vi "Auto Loop.vi"(8 "error in":errorcluster, 10 "semaphore":T3, 11 "Queues in":T10) -> (0 "error out":errorcluster, 2 "semaphore out":T3)   [LabVIEW 2017]
doc: "This is the loop that handles the testing algorithms\n\n--------------\nv0.1:\n\n- Updated Printer"
uses:
  support/Message Queue/All Message Queues.ctl
  support/Message Queue/Message Cluster.ctl
  controls/Model Name.ctl
  controls/Auto States v0.2.ctl
  controls/All Specs.ctl
  controls/Specifications.ctl
  controls/Results Cluster.ctl
  controls/AC Results.ctl
  controls/Update Measurements.ctl
  <vilib>/Platform/TimedLoop/XDataNode/timing_clust.ctl
  <vilib>/Platform/TimedLoop/XDataNode/nitl_modes.ctl
  <vilib>/Platform/TimedLoop/XDataNode/wakeup.ctl
  controls/Towerlight.ctl
  support/Message Queue/Enqueue Message (Single).vi
  GV/All Inputs.vi
  support/GV/Towerlight GV.vi
  GV/TEST GV/Test auto state machine.vi
  <vilib>/platform/TimedLoop/XDataNode/XDataNode.xnode
  controls/FGV DO.ctl
  <vilib>/Platform/TimedLoop/XDataNode/XDNodeRunTimeDep.lvlib
  support/Message Queue/Message Queue.lvlib
panel:
  out "Results 2":T1
  out "TS Status 2":cluster{"Status":string, "Elapsed Time":dbl}
  out "Results Cluster out 2":T2
  out "Graph 2":dbl[][](array[numeric])
  out "cycle time 2":u32
  out "Specs":T4={"LH"={"Go Up"={"Min Speed"=120.0, "Max Speed"=10.0, "Min Time"=1.82, "Max Time"=3.7, "Min Run Current"=0.0, "Max Run Current"=10.0, "Min Stall Current"=0.0, "Max Stall Current"=25.0, "Min Stall Force"=170.0, "Max Stall Force"=320.0, "Min Stroke"=170.0, "Max Stroke"=320.0}, "Go Down"={"Min Speed"=10.0, "Max Speed"=250.0, "Min Travel Time"=1.82, "Max Travel Time"=3.7, "Min Run Current"=0.0, "Max Run Current"=10.0}, "Shipping"={"Min Distance"=150.0, "Max Distance"=300.0, "Setpoint"=5.0}, "Anti-Pinch"={"Min Force"=5.0, "Max Force"=15.0}}, "RH"={"Go Up"={"Min Speed"=120.0, "Max Speed"=10.0, "Min Time"=1.82, "Max Time"=3.7, "Min Run Current"=0.0, "Max Run Current"=10.0, "Min Stall Current"=0.0, "Max Stall Current"=25.0, "Min Stall Force"=170.0, "Max Stall Force"=320.0, "Min Stroke"=170.0, "Max Stroke"=320.0}, "Go Down"={"Min Speed"=10.0, "Max Speed"=250.0, "Min Travel Time"=1.82, "Max Travel Time"=3.7, "Min Run Current"=0.0, "Max Run Current"=10.0}, "Shipping"={"Min Distance"=150.0, "Max Distance"=300.0, "Setpoint"=5.0}, "Anti-Pinch"={"Min Force"=5.0, "Max Force"=15.0}}, "W 601 FR RH Std"={"Go Up"={"Min Speed"=10.0, "Max Speed"=250.0, "Min Time"=0.5, "Max Time"=4.3, "Min Run Current"=0.0, "Max Run Current"=10.0, "Min Stall Current"=0.0, "Max Stall Current"=25.0, "Min Stall Force"=170.0, "Max Stall Force"=320.0, "Min Stroke"=254.4, "Max Stroke"=270.4}, "Go Down"={"Min Speed"=10.0, "Max Speed"=250.0, "Min Travel Time"=0.5, "Max Travel Time"=4.3, "Min Run Current"=0.0, "Max Run Current"=10.0}, "Shipping"={"Min Distance"=5.0, "Max Distance"=15.0, "Setpoint"=5.0}, "Anti-Pinch"={"Min Force"=5.0, "Max Force"=15.0}}, "W 601 FR LH Std"={"Go Up"={"Min Speed"=10.0, "Max Speed"=250.0, "Min Time"=0.5, "Max Time"=4.3, "Min Run Current"=0.0, "Max Run Current"=10.0, "Min Stall Current"=0.0, "Max Stall Current"=25.0, "Min Stall Force"=170.0, "Max Stall Force"=320.0, "Min Stroke"=254.4, "Max Stroke"=270.4}, "Go Down"={"Min Speed"=10.0, "Max Speed"=250.0, "Min Travel Time"=0.5, "Max Travel Time"=4.3, "Min Run Current"=0.0, "Max Run Current"=10.0}, "Shipping"={"Min Distance"=5.0, "Max Distance"=15.0, "Setpoint"=5.0}, "Anti-Pinch"={"Min Force"=5.0, "Max Force"=15.0}}, "W 601 RR RH Std"={"Go Up"={"Min Speed"=10.0, "Max Speed"=250.0, "Min Time"=0.5, "Max Time"=4.3, "Min Run Current"=0.0, "Max Run Current"=10.0, "Min Stall Current"=0.0, "Max Stall Current"=25.0, "Min Stall Force"=170.0, "Max Stall Force"=320.0, "Min Stroke"=254.4, "Max Stroke"=270.4}, "Go Down"={"Min Speed"=10.0, "Max Speed"=250.0, "Min Travel Time"=0.5, "Max Travel Time"=4.3, "Min Run Current"=0.0, "Max Run Current"=10.0}, "Shipping"={"Min Distance"=5.0, "Max Distance"=15.0, "Setpoint"=5.0}, "Anti-Pinch"={"Min Force"=5.0, "Max Force"=15.0}}, "W 601 RR LH Std"={"Go Up"={"Min Speed"=10.0, "Max Speed"=250.0, "Min Time"=0.5, "Max Time"=4.3, "Min Run Current"=0.0, "Max Run Current"=10.0, "Min Stall Current"=0.0, "Max Stall Current"=25.0, "Min Stall Force"=170.0, "Max Stall Force"=320.0, "Min Stroke"=254.4, "Max Stroke"=270.4}, "Go Down"={"Min Speed"=10.0, "Max Speed"=250.0, "Min Travel Time"=0.5, "Max Travel Time"=4.3, "Min Run Current"=0.0, "Max Run Current"=10.0}, "Shipping"={"Min Distance"=5.0, "Max Distance"=15.0, "Setpoint"=5.0}, "Anti-Pinch"={"Min Force"=5.0, "Max Force"=15.0}}, "W 601 FR RH AP"={"Go Up"={"Min Speed"=10.0, "Max Speed"=250.0, "Min Time"=0.5, "Max Time"=4.3, "Min Run Current"=0.0, "Max Run Current"=10.0, "Min Stall Current"=0.0, "Max Stall Current"=25.0, "Min Stall Force"=170.0, "Max Stall Force"=320.0, "Min Stroke"=254.4, "Max Stroke"=270.4}, "Go Down"={"Min Speed"=10.0, "Max Speed"=250.0, "Min Travel Time"=0.5, "Max Travel Time"=4.3, "Min Run Current"=0.0, "Max Run Current"=10.0}, "Shipping"={"Min Distance"=5.0, "Max Distance"=15.0, "Setpoint"=5.0}, "Anti-Pinch"={"Min Force"=5.0, "Max Force"=15.0}}, "W 601 FR LH AP"={"Go Up"={"Min Speed"=10.0, "Max Speed"=250.0, "Min Time"=0.5, "Max Time"=4.3, "Min Run Current"=0.0, "Max Run Current"=10.0, "Min Stall Current"=0.0, "Max Stall Current"=25.0, "Min Stall Force"=170.0, "Max Stall Force"=320.0, "Min Stroke"=254.4, "Max Stroke"=270.4}, "Go Down"={"Min Speed"=10.0, "Max Speed"=250.0, "Min Travel Time"=0.5, "Max Travel Time"=4.3, "Min Run Current"=0.0, "Max Run Current"=10.0}, "Shipping"={"Min Distance"=5.0, "Max Distance"=15.0, "Setpoint"=5.0}, "Anti-Pinch"={"Min Force"=5.0, "Max Force"=15.0}}, "W 601 RR RH AP"={"Go Up"={"Min Speed"=10.0, "Max Speed"=250.0, "Min Time"=0.5, "Max Time"=4.3, "Min Run Current"=0.0, "Max Run Current"=10.0, "Min Stall Current"=0.0, "Max Stall Current"=25.0, "Min Stall Force"=170.0, "Max Stall Force"=320.0, "Min Stroke"=254.4, "Max Stroke"=270.4}, "Go Down"={"Min Speed"=10.0, "Max Speed"=250.0, "Min Travel Time"=0.5, "Max Travel Time"=4.3, "Min Run Current"=0.0, "Max Run Current"=10.0}, "Shipping"={"Min Distance"=5.0, "Max Distance"=15.0, "Setpoint"=5.0}, "Anti-Pinch"={"Min Force"=5.0, "Max Force"=15.0}}, "W 601 RR LH AP"={"Go Up"={"Min Speed"=10.0, "Max Speed"=250.0, "Min Time"=0.5, "Max Time"=4.3, "Min Run Current"=0.0, "Max Run Current"=10.0, "Min Stall Current"=0.0, "Max Stall Current"=25.0, "Min Stall Force"=170.0, "Max Stall Force"=320.0, "Min Stroke"=254.4, "Max Stroke"=270.4}, "Go Down"={"Min Speed"=10.0, "Max Speed"=250.0, "Min Travel Time"=0.5, "Max Travel Time"=4.3, "Min Run Current"=0.0, "Max Run Current"=10.0}, "Shipping"={"Min Distance"=5.0, "Max Distance"=15.0, "Setpoint"=5.0}, "Anti-Pinch"={"Min Force"=5.0, "Max Force"=15.0}}}
  out "Counts":T6
  out "AC State":T7
  in  "Initial Data":T9={"Model Name"=enum."W 501 FLH Std.", "ID"="ID", "Shift"=""}
  in  "Exit":bool
  out "Period":i64
  in  "Run Auto?":bool
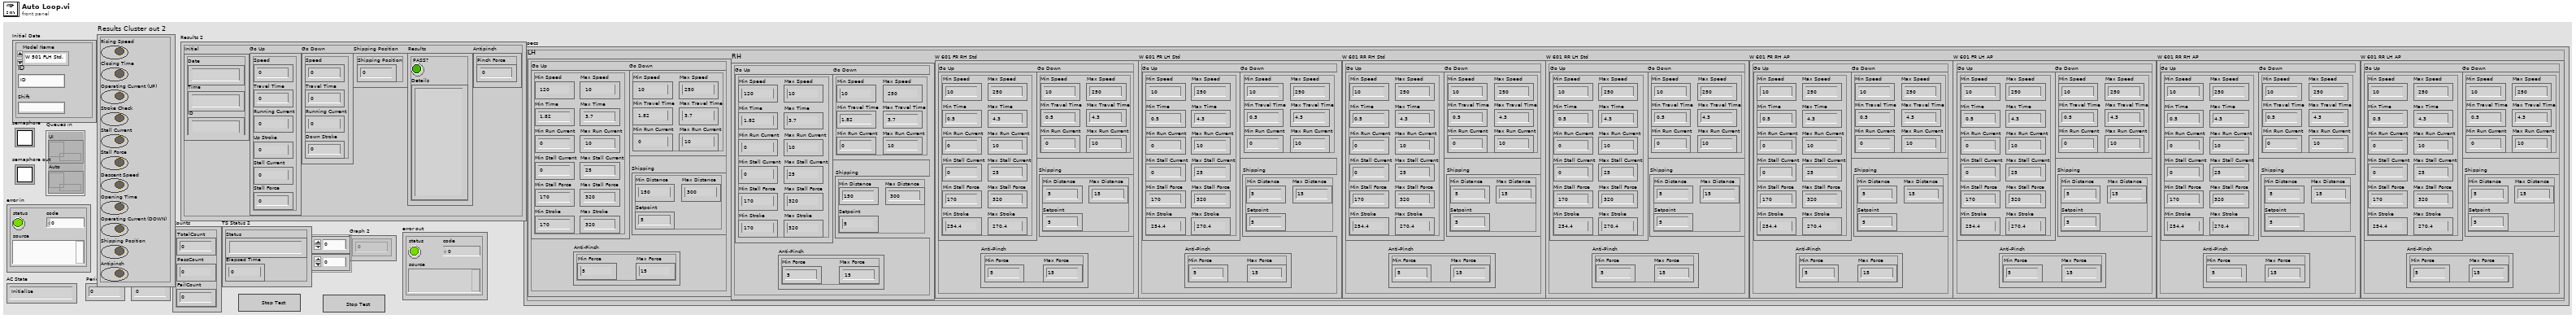
[diagram p1: front panel]
types:
  T1 = typedef "AC Results.ctl" = cluster{"Initial":cluster{"Date":string, "Time":string, "ID":string}, "Go Up":cluster{"Speed":dbl, "Travel Time":dbl, "Running Current":dbl, "Up Stroke":dbl, "Stall Current":dbl, "Stall Force":dbl}, "Go Down":cluster{"Speed":dbl, "Travel Time":dbl, "Running Current":dbl, "Down Stroke":dbl}, "Shipping Position":cluster{"Shipping Position":dbl}, "Results":cluster{"PASS?":bool, "Details":string}, "Antipinch":cluster{"Pinch Force":dbl}}
  T2 = typedef "Results Cluster.ctl" = cluster{"Rising Speed":bool, "Closing Time":bool, "Operating Current (UP)":bool, "Stroke Check":bool, "Stall Current":bool, "Stall Force":bool, "Descent Speed":bool, "Opening Time":bool, "Operating Current (DOWN)":bool, "Shipping Position":bool, "Antipinch":bool}
  T3 = typedef "Semaphore RefNum" = refnum<k1>
  T4 = typedef "All Specs.ctl" = cluster{"LH":T5, "RH":T5, "W 601 FR RH Std":T5, "W 601 FR LH Std":T5, "W 601 RR RH Std":T5, "W 601 RR LH Std":T5, "W 601 FR RH AP":T5, "W 601 FR LH AP":T5, "W 601 RR RH AP":T5, "W 601 RR LH AP":T5}
  T5 = typedef "Specifications.ctl" = cluster{"Go Up":cluster{"Min Speed":dbl, "Max Speed":dbl, "Min Time":dbl, "Max Time":dbl, "Min Run Current":dbl, "Max Run Current":dbl, "Min Stall Current":dbl, "Max Stall Current":dbl, "Min Stall Force":dbl, "Max Stall Force":dbl, "Min Stroke":dbl, "Max Stroke":dbl}, "Go Down":cluster{"Min Speed":dbl, "Max Speed":dbl, "Min Travel Time":dbl, "Max Travel Time":dbl, "Min Run Current":dbl, "Max Run Current":dbl}, "Shipping":cluster{"Min Distance":dbl, "Max Distance":dbl, "Setpoint":dbl}, "Anti-Pinch":cluster{"Min Force":dbl, "Max Force":dbl}}
  T6 = cluster{"TotalCount":u16, "PassCount":u16, "FailCount":u16}
  T7 = typedef "Auto States v0.2.ctl" = enum16{"Initialize", "Check Pressure", "Check EStop", "Check Reject Door ", "Check ReadyCondition", "Wait to Home", "Declamping", "Loadcell CYL to Home", "Wait for Part Presence", "Wait for Hands-Off", "Clamp", "Wait for Load Engage", "Wait for Start", "Test Sequencer", "Log & Print", "check for pass or fail", "Result", "Wait for Reject Door Open", "Wait for Reject 2 OFF", "Wait for Reject 2 ON", "Wait for Reject 1 OFF", "Wait for Reject 1 ON", "Wait for Reject Door Close"}
  T8 = typedef "Model Name.ctl" = enum16{"W 501 FLH Std.", "W 501 FRH Std.", "W 601 FR RH Std", "W 601 FR LH Std", "W 601 RR RH Std", "W 601 RR LH Std", "W 601 FR RH AP", "W 601 FR LH AP", "W 601 RR RH AP", "W 601 RR LH AP"}
  T9 = cluster{"Model Name":T8, "ID":string, "Shift":string}
  T10 = typedef "Message Queue.lvlib/All Message Queues.ctl" = cluster{"UI":refnum<queue>, "Auto":refnum<queue>}
  T11 = cluster{"AI":refnum<k21>, "DI":refnum<k21>, "Counter":refnum<k21>}
  T12 = typedef "Towerlight.ctl" = enum16{"Idle", "Error", "Attention", "Running", "Maintenance", "Fail"}
  T13 = typedef "FGV DO.ctl" = enum16{"Initialize", "Start Task", "Clamping", "Load CYL", "Contactors", "Loadcell CYL", "BSL", "Read DO", "Clear Tasks", "Clear Task"}
  T14 = typedef "XDNodeRunTimeDep.lvlib/timing_clust.ctl" = cluster{"Expected End [f-1]":u64, "Actual End [f-1]":u64, "Finished Late? [f-1]":bool, "Expected End [i-1]":u64, "Actual End [i-1]":u64, "Finished Late? [i-1]":bool, "Expected Start [i]":u64, "Actual Start [i]":u64, "Expected Start [f]":u64, "Actual Start [f]":u64, "Source Name":string, "Structure Name":string, "Period":i64, "Deadline":i64, "Offset":i64, "Start":i64, "Priority":i32, "Timeout":i32, "Mode":T15, "Wakeup Reason":T16, "Error":errorcluster, "Source Type":string, "Secondary Source Type":string, "Global End Time":u64, "Global Start Time":u64, "Frame Duration":u64, "Iteration Duration":u64, "Assigned CPU":i32, "I/O Scan Engine Mode":u32}
  T15 = typedef "XDNodeRunTimeDep.lvlib/nitl_modes.ctl" = enum32{"No Change", "Process missed periods, maintain original phase", "Discard missed periods, maintain original phase", "Process missed periods, ignore original phase", "Discard missed periods, ignore original phase"}
  T16 = typedef "XDNodeRunTimeDep.lvlib/wakeup.ctl" = enum32{"Normal", "Aborted", "Asynchronous wakeup", "Timing source error", "Timed loop error", "Timeout"}
  T17 = typedef "All Inputs.ctl" = cluster{"DI":cluster{"Machine ON":bool, "E-Stop":bool, "Pressure":bool, "Start":bool, "Safety Curtain":bool, "RS Load UP Rear":bool, "RS Load UP Front":bool, "RS Load DN Rear":bool, "RS Load DN Front":bool, "RS Loadcell Rear":bool, "RS Loadcell Front":bool, "Reject Sensor 1":bool, "Reject Sensor 2":bool, "Door SW Reject":bool}, "AI":cluster{"Force":dbl[], "Stroke":dbl[], "CurrentMon":dbl[]}, "SACB Inputs":T18}
  T18 = typedef "SACB DI.ctl" = cluster{"RS ClampTop Front":bool, "RS ClampBottom Front":bool, "RS ClampMotorLH Front":bool, "RS ClampMotorRH Front":bool, "IPS PartPresenceTop LH":bool, "IPS PartPresenceBottom LH":bool, "IPS PartPresenceTop RH":bool, "IPS PartPresenceBottom RH":bool, "IPS LoadEngaged 1":bool, "IPS LoadEngaged 2":bool, "IPS LoadEngaged 3":bool, "C11":bool, "C12":bool, "C13":bool, "C14":bool, "C15":bool}
  T19 = cluster{"Pressure":bool, "E Stop":bool, "Reject Door":bool, "Ready Condition":bool, " Home":bool, " De Clamb":bool, " Load Cell":bool, " Part Presence":bool, " Hands Off":bool, "Clamp":bool, " Load engage":bool, "Wait Start":bool, "Test Sequencer":bool}
  T20 = typedef "Update Measurements.ctl" = cluster{"Results":T1, "TS Status":cluster{"Status":string, "Elapsed Time":dbl}, "Counts":cluster{"TotalCount":u16, "PassCount":u16, "FailCount":u16}, "AC Graph":cluster{"X":dbl, "Y":dbl}[], "Total Time":dbl, "Testing Time (s)":dbl, "Graph":dbl[][], "signal out":waveform(dbl)}
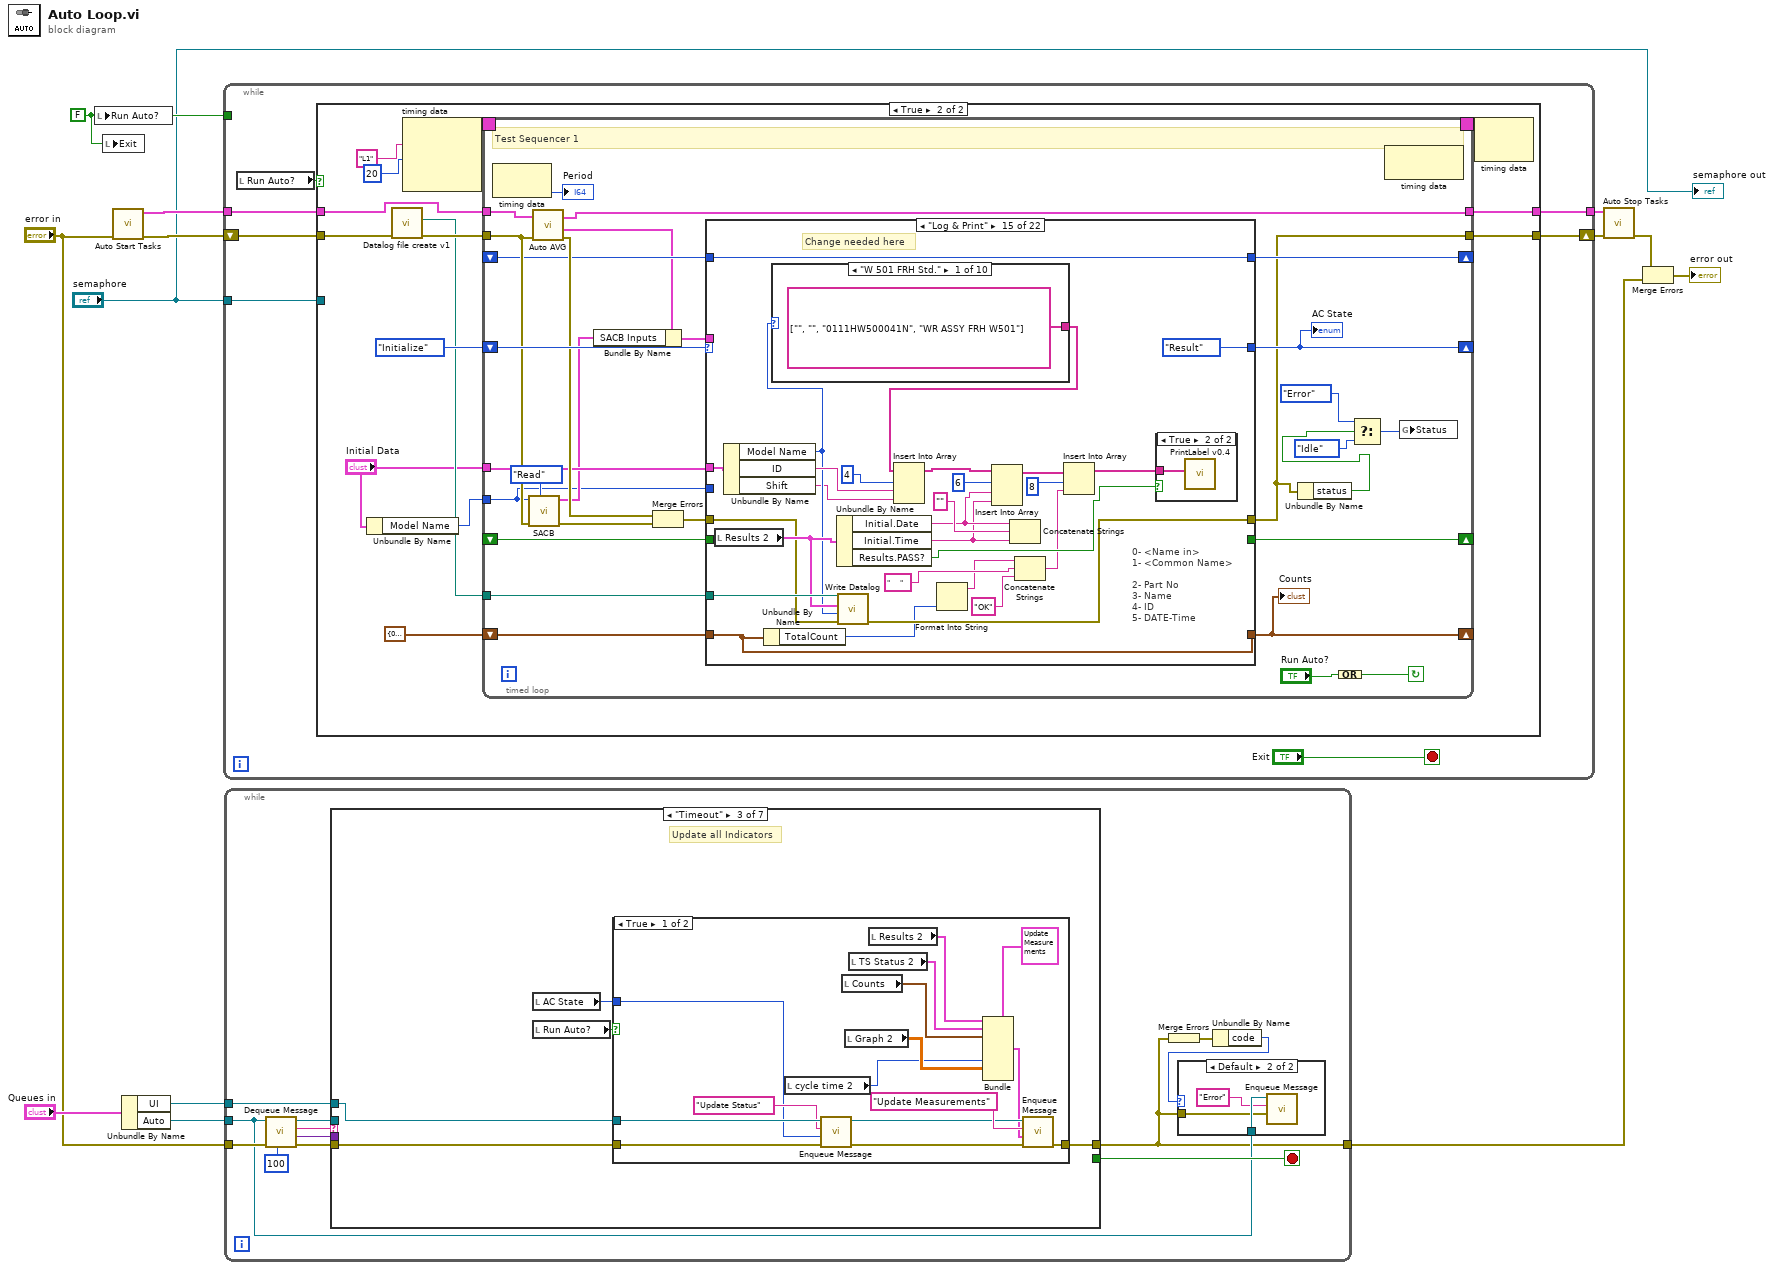
[diagram p0: block diagram]
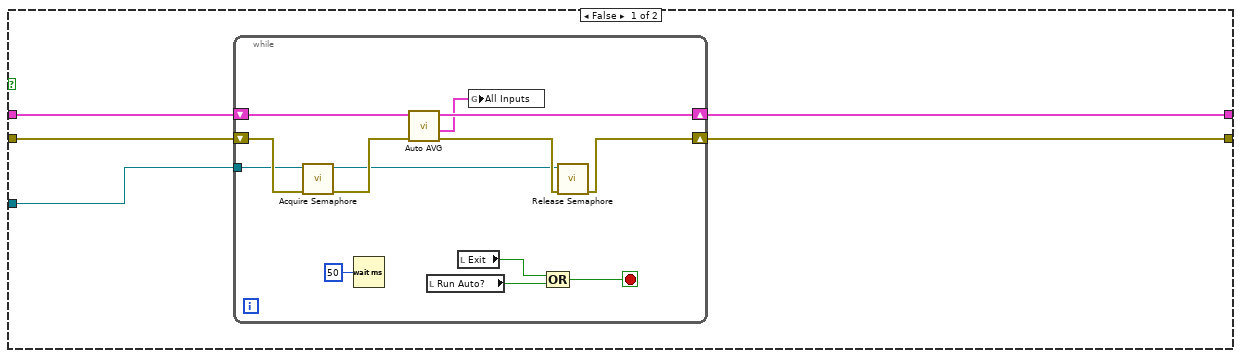
[diagram p2: hidden frame]
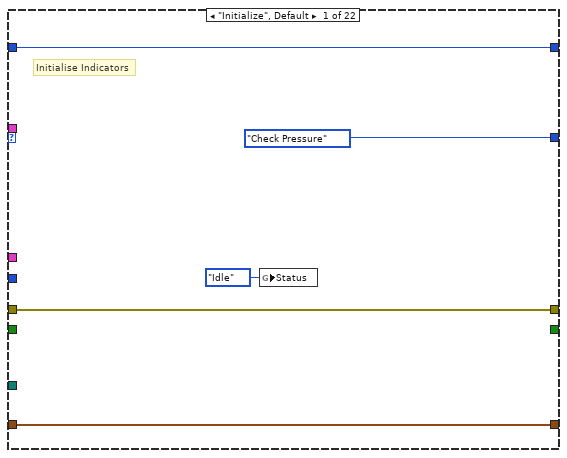
[diagram p3: hidden frame]
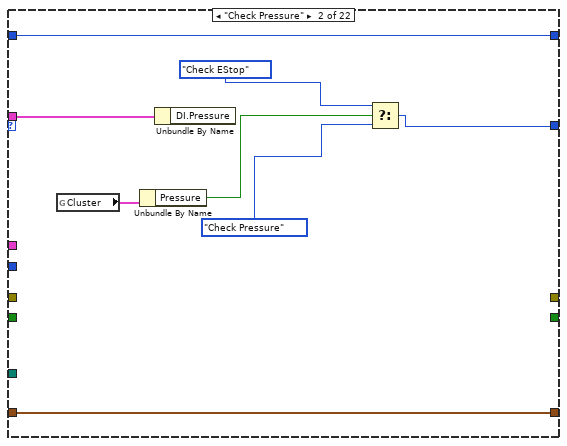
[diagram p4: hidden frame]
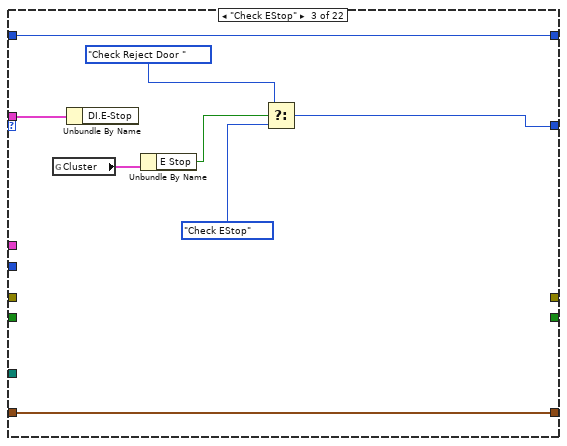
[diagram p5: hidden frame]
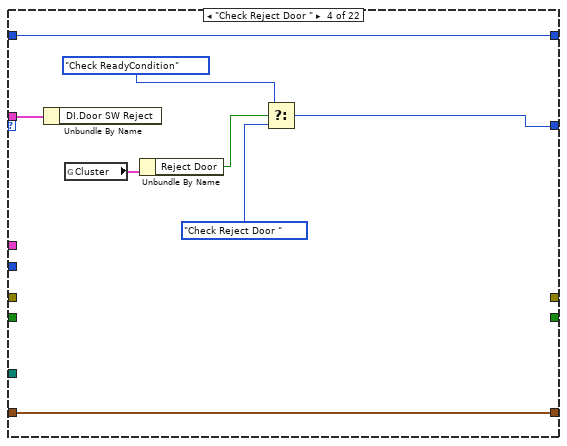
[diagram p6: hidden frame]
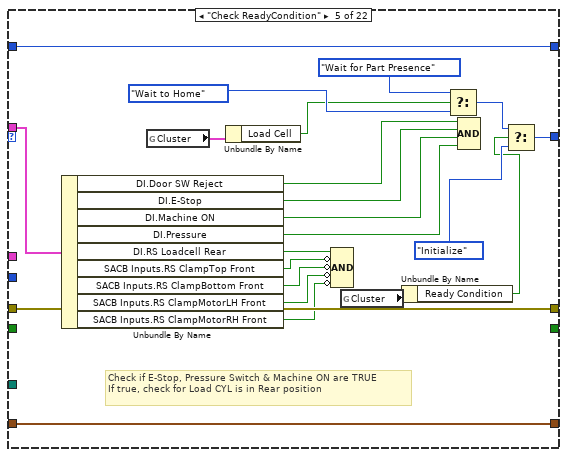
[diagram p7: hidden frame]
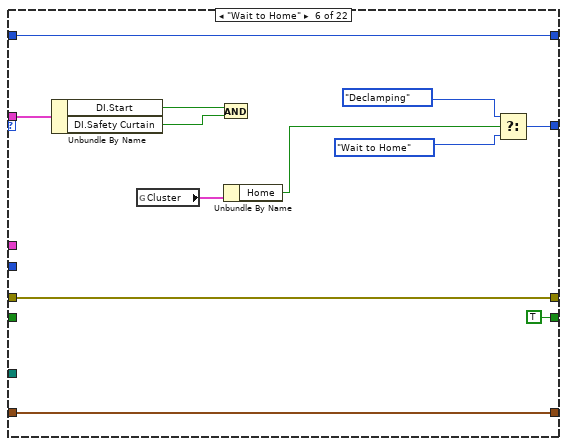
[diagram p8: hidden frame]
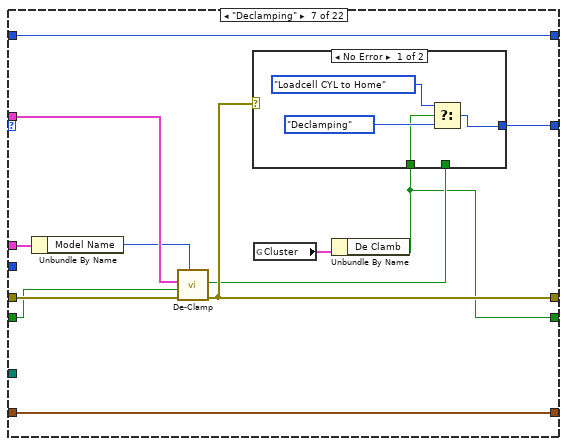
[diagram p9: hidden frame]
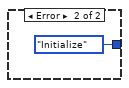
[diagram p10: hidden frame]
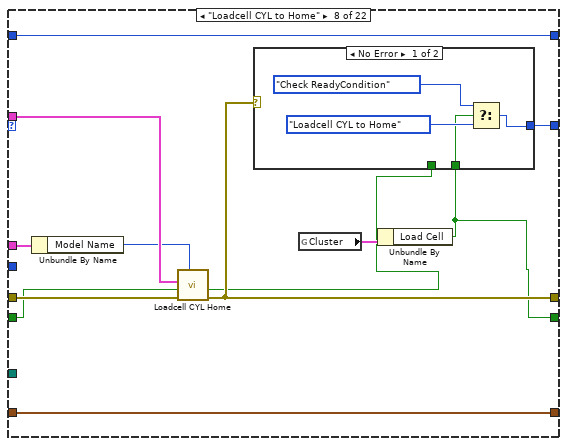
[diagram p11: hidden frame]
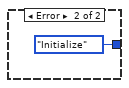
[diagram p12: hidden frame]
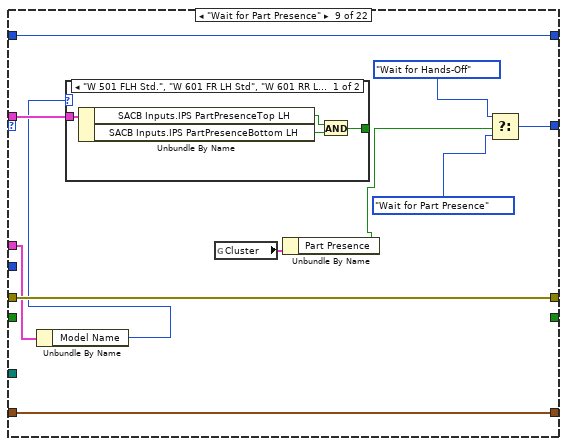
[diagram p13: hidden frame]
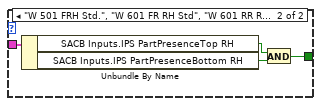
[diagram p14: hidden frame]
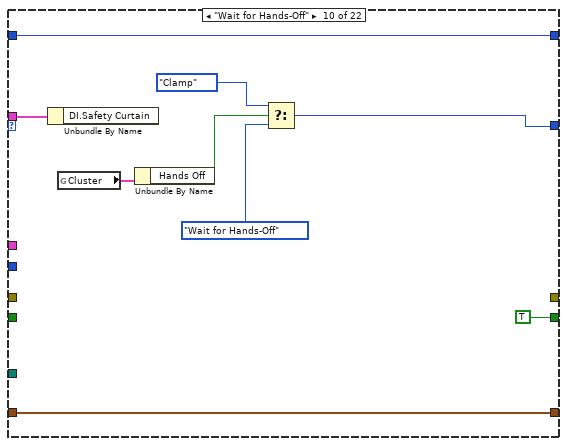
[diagram p15: hidden frame]
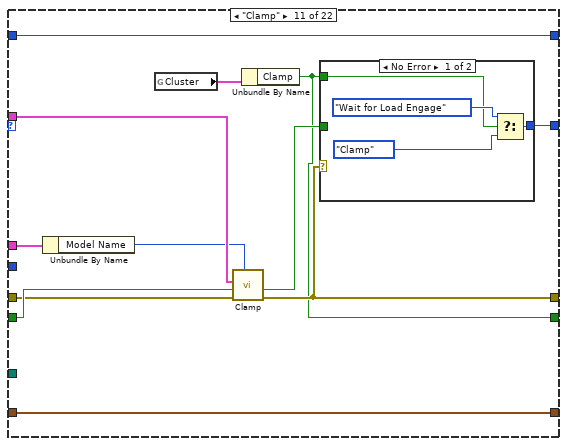
[diagram p16: hidden frame]
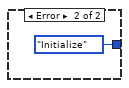
[diagram p17: hidden frame]
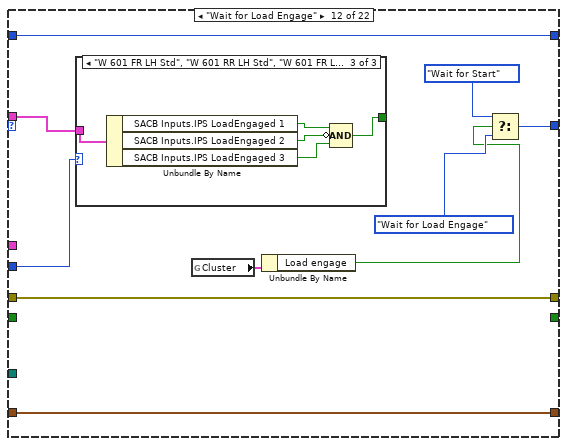
[diagram p18: hidden frame]
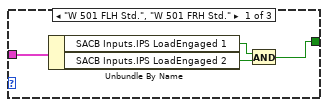
[diagram p19: hidden frame]
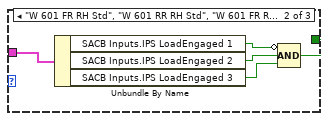
[diagram p20: hidden frame]
diagram:
  w8 = FALSE ("Run Auto?")
  n1 = local write "Run Auto?"(w8) -> ()
  n2 = local write "Exit"(w8) -> ()
  n3 = call "Auto Start Tasks.vi"("error in"="error in") -> ("error out"=w6:errorcluster, "All Input Tasks"=w7:T11)  [unwired: 9 in]
  n4 = Unbundle By Name("Queues in") -> ("UI"=w9:refnum<queue>, "Auto"=w12:refnum<queue>)
  n5 = while {
    shift-right: [w15] -> w3
    shift-left: w6 -> [w17]
    tunnel: w8 -> [_]
    tunnel: w7 -> [w18]
    tunnel: [w16] -> w5
    tunnel: "semaphore" -> [w14]
    stop <- "Exit" stop-if-true
    n6 = local read "Run Auto?"() -> (w19:bool)
    n7 = case shown="True" w19 {
      tunnel: [w23 w43] -> w15
      tunnel: w17 -> [w24 w41]
      tunnel: w18 -> [w25 w44]
      tunnel: [w22 w42] -> w16
      tunnel: w14 -> [w21 _]
      frame False {
        n8 = while {
          shift-right: [w36] -> w22
          shift-left: w25 -> [w37]
          shift-right: [w28] -> w23
          shift-left: w24 -> [w31]
          tunnel: w21 -> [w26]
          stop <- w34 stop-if-true
          n9 = call <vilib>:"Acquire Semaphore.vi"("error in (no error)"=w31, "semaphore"=w26) -> ("error out"=w30:errorcluster, "semaphore out"=w27:T3)  [unwired: 3 in, 1 out]
          n10 = Wait (ms)(milliseconds to wait=u32 50) -> ()  [unwired: 1 out]
          n11 = call "Auto AVG.vi"("error in"=w30, "All Input Tasks in"=w37) -> ("error out"=w29:errorcluster, "All Inputs cluster"=w32:T17, "All Input Tasks out"=w36:T11)  [unwired: 7 in]
          n12 = local read "Run Auto?"() -> (w35:bool)
          n13 = local read "Exit"() -> (w33:bool)
          n14 = global write "All Inputs.vi" "All Inputs"(w32) -> ()
          n15 = Compound Arithmetic op=OR(w33, w35) -> (w34:bool)
          n16 = call <vilib>:"Release Semaphore.vi"("error in (no error)"=w29, "semaphore"=w27) -> ("error out"=w28:errorcluster)  [unwired: 4 in, 1 out]
        }
      }
      frame True {
        n17 = Unbundle By Name("Initial Data") -> ("Model Name"=w39:T8)
        n18 = call "Datalog file create v1.vi"("error in (no error)"=w41) -> ("error out"=w46:errorcluster, "File path out"=w45:path)  [unwired: 9 in]
        n19 = node-c288("L1" ("Structure Name"), i64 20 ("Period")) -> (w52:T14)  [unwired: 1 in]
        n20 = timed-loop {
          timing: w52 -> [_]
          timing-out: [_] -> w51
          tunnel: [w54] -> w42
          shift-right: [w76] -> _
          shift-left: Auto_States_v0.2."Initialize" -> [w77]
          tunnel: [w61] -> w43
          tunnel: "Initial Data" -> [w72]
          shift-right: [w73] -> _
          shift-left: _ -> [w74]
          shift-right: [w70] -> _
          shift-left: T6 {"TotalCount"=0, "PassCount"=0, "FailCount"=0} ("Counts") -> [w71]
          tunnel: w45 -> [w69]
          tunnel: w46 -> [w67]
          tunnel: w44 -> [w68]
          shift-right: [w63] -> _
          shift-left: _ -> [w62]
          tunnel: w39 -> [w53]
          stop <- w80 continue-if-true
          # "Test Sequencer 1"
          n21 = node-c288() -> (→"Period":i64)  [unwired: 1 in]
          n22 = call "SACB.vi"("Command"=enum16{"Create", "Read", "Close"}."Read", "Error In"=w67, "Model Name"=w53) -> ("Error Out"=w66:errorcluster, "Digital Inputs"=w56:T18)  [unwired: 6 in, 1 out]
          n23 = call "Auto AVG.vi"("error in"=w67, "All Input Tasks in"=w68) -> ("error out"=w75:errorcluster, "All Inputs cluster"=w55:T17, "All Input Tasks out"=w54:T11)  [unwired: 7 in]
          n24 = Bundle By Name(cluster=w55, "SACB Inputs"=w56) -> (w65:T17)
          n25 = Merge Errors(w75, w66) -> (w78:errorcluster)
          n26 = case shown="\"Log & Print\"" w77 {
            tunnel: w78 -> [w85 _ _ _ w132 w140 w153 w170 w186 _ w216 w231 w263 w301 w318 w350 w400 w409 w417 w425 w433 w449]
            tunnel: [Auto_States_v0.2."Check Pressure" w91 w99 w107 w127 w141 w156 w173 w187 w203 w218 w232 w264 w297 Auto_States_v0.2."Result" w351 w403 w412 w420 w428 w436 w439] -> w76
            tunnel: [w85 _ _ _ w132 w140 w148 w165 w186 _ w211 w231 w263 w293 w317 w350 w400 w409 w417 w425 w433 w449] -> w61
            tunnel: w72 -> [_ _ _ _ _ _ w151 w168 w183 _ w214 _ w259 w281 w328 w349 _ _ _ _ _ _]
            tunnel: w74 -> [_ _ _ _ _ _ w149 w166 _ _ w217 _ _ w300 _ _ _ _ _ _ _ _]
            tunnel: [_ _ _ _ _ TRUE ("Completed? out") w145 w163 _ TRUE ("Completed? out") w207 _ w248 w280 _ _ _ _ _ _ _ _] -> w73
            tunnel: w71 -> [w83 w94 w102 w110 w131 w139 w155 w172 w185 w206 w212 w230 w262 w292 w313 w348 w404 w413 w421 w429 w437 w450]
            tunnel: [w83 w94 w102 w110 w131 w139 w155 w172 w185 w206 w212 w230 w262 w291 w313 w348 w404 w413 w421 w429 w437 w450] -> w70
            tunnel: w69 -> [_ _ _ _ _ _ _ _ _ _ _ _ _ _ w321 _ _ _ _ _ _ _]
            tunnel: w65 -> [_ w90 w98 w106 w130 w138 w152 w169 w184 w202 w215 w229 w254 w289 _ w345 w398 w407 w415 w423 w431 w447]
            tunnel: [w82 w89 w97 w105 w125 w137 w154 w171 w181 w200 w210 w228 w256 w282 w316 w347 w399 w408 w416 w424 w432 w448] -> w63
            tunnel: w62 -> [w82 w89 w97 w105 w125 w137 w154 w171 w181 w200 w210 w228 _ w282 w316 w347 w399 w408 w416 w424 w432 w448]
            tunnel: w53 -> [_ _ _ _ _ _ _ _ _ _ _ w226 _ _ _ _ _ _ _ _ _ _]
            frame "Initialize", Default {
              # "Initialise Indicators"
              n27 = global write "Towerlight GV.vi" "Status"(Towerlight."Idle" ("Status")) -> ()
            }
            frame "Check Pressure" {
              n28 = global read "Test auto state machine.vi" "Cluster"() -> (w88:T19)
              n29 = Unbundle By Name(w88) -> ("Pressure"=w87:bool)
              n30 = Unbundle By Name(w90) -> ()  [unwired: 1 out]
              n31 = Select(t=Auto_States_v0.2."Check EStop", s=w87, f=Auto_States_v0.2."Check Pressure") -> (s? t:f=w91:T7)
            }
            frame "Check EStop" {
              n32 = global read "Test auto state machine.vi" "Cluster"() -> (w96:T19)
              n33 = Unbundle By Name(w98) -> ()  [unwired: 1 out]
              n34 = Unbundle By Name(w96) -> ("E Stop"=w95:bool)
              n35 = Select(t=Auto_States_v0.2."Check Reject Door ", s=w95, f=Auto_States_v0.2."Check EStop") -> (s? t:f=w99:T7)
            }
            frame "Check Reject Door " {
              n36 = Unbundle By Name(w106) -> ()  [unwired: 1 out]
              n37 = global read "Test auto state machine.vi" "Cluster"() -> (w104:T19)
              n38 = Unbundle By Name(w104) -> ("Reject Door"=w103:bool)
              n39 = Select(t=Auto_States_v0.2."Check ReadyCondition", s=w103, f=Auto_States_v0.2."Check Reject Door ") -> (s? t:f=w107:T7)
            }
            frame "Check ReadyCondition" {
              # "Check if E-Stop, Pressure Switch & Machine ON are TRUE\nIf true, check for Load CYL is in Rear position"
              n40 = Unbundle By Name(w130) -> ("DI.Door SW Reject"=w115:bool, "DI.E-Stop"=w129:bool, "DI.Machine ON"=w128:bool, "DI.Pressure"=w124:bool, "DI.RS Loadcell Rear"=w123:bool, "SACB Inputs.RS ClampTop Front"=w122:bool, "SACB Inputs.RS ClampBottom Front"=w121:bool, "SACB Inputs.RS ClampMotorLH Front"=w120:bool, "SACB Inputs.RS ClampMotorRH Front"=w119:bool)
              n41 = global read "Test auto state machine.vi" "Cluster"() -> (w114:T19)
              n42 = Unbundle By Name(w114) -> ("Load Cell"=w111:bool)
              n43 = Compound Arithmetic op=AND(w123, invert w122, invert w121, invert w120, invert w119) -> ()  [unwired: 1 out]
              n44 = global read "Test auto state machine.vi" "Cluster"() -> (w113:T19)
              n45 = Unbundle By Name(w113) -> ("Ready Condition"=w112:bool)
              n46 = Select(t=Auto_States_v0.2."Wait for Part Presence" ("f"), s=w111, f=Auto_States_v0.2."Wait to Home") -> (s? t:f=w117:T7)
              n47 = Compound Arithmetic op=AND(w115, w129, w128, w124) -> ()  [unwired: 1 out]
              n48 = Select(t=w117, s=w112, f=Auto_States_v0.2."Initialize") -> (s? t:f=w127:T7)
            }
            frame "Wait to Home" {
              n49 = Unbundle By Name(w138) -> ("DI.Start"=w144:bool, "DI.Safety Curtain"=w136:bool)
              n50 = global read "Test auto state machine.vi" "Cluster"() -> (w134:T19)
              n51 = And(x=w144, y=w136) -> ()  [unwired: 1 out]
              n52 = Unbundle By Name(w134) -> ("Home"=w133:bool)
              n53 = Select(t=Auto_States_v0.2."Declamping", s=w133, f=Auto_States_v0.2."Wait to Home") -> (s? t:f=w141:T7)
            }
            frame "Declamping" {
              n54 = Unbundle By Name(w151) -> ("Model Name"=w150:T8)
              n55 = call "De-Clamp.vi"("Model Name"=w150, "Error In"=w153, "Intialize?"=w149, "Inputs"=w152) -> ("error out"=w148:errorcluster, "Completed"=w146:bool)  [unwired: 5 in, 1 out]
              n56 = global read "Test auto state machine.vi" "Cluster"() -> (w147:T19)
              n57 = Unbundle By Name(w147) -> ("De Clamb"=w145:bool)
              n58 = case shown="No Error" w148 {
                tunnel: [w158 Auto_States_v0.2."Initialize"] -> w156
                tunnel: w145 -> [w157 _]
                tunnel: w146 -> [_ _]
                frame No Error {
                  n59 = Select(t=Auto_States_v0.2."Loadcell CYL to Home", s=w157, f=Auto_States_v0.2."Declamping") -> (s? t:f=w158:T7)
                }
                frame Error {
                }
              }
            }
            frame "Loadcell CYL to Home" {
              n60 = Unbundle By Name(w168) -> ("Model Name"=w167:T8)
              n61 = call "Loadcell CYL Home.vi"("Model Name"=w167, "Error In"=w170, "Intialize?"=w166, "Inputs"=w169) -> ("error out"=w165:errorcluster, "Completed"=w162:bool)  [unwired: 5 in, 1 out]
              n62 = global read "Test auto state machine.vi" "Cluster"() -> (w164:T19)
              n63 = Unbundle By Name(w164) -> ("Load Cell"=w163:bool)
              n64 = case shown="No Error" w165 {
                tunnel: [w175 Auto_States_v0.2."Initialize"] -> w173
                tunnel: w163 -> [w174 _]
                tunnel: w162 -> [_ _]
                frame No Error {
                  n65 = Select(t=Auto_States_v0.2."Check ReadyCondition", s=w174, f=Auto_States_v0.2."Loadcell CYL to Home") -> (s? t:f=w175:T7)
                }
                frame Error {
                }
              }
            }
            frame "Wait for Part Presence" {
              n66 = Unbundle By Name(w183) -> ("Model Name"=w182:T8)
              n67 = case shown="\"W 501 FLH Std.\", \"W 601 FR LH Std\", \"W 601 RR LH Std\", \"W 601 FR LH AP\", \"W 601 RR LH AP\"" w182 {
                tunnel: w184 -> [w193 w197]
                tunnel: [w190 w194] -> _
                frame "W 501 FLH Std.", "W 601 FR LH Std", "W 601 RR LH Std", "W 601 FR LH AP", "W 601 RR LH AP" {
                  n68 = Unbundle By Name(w193) -> ("SACB Inputs.IPS PartPresenceTop LH"=w191:bool, "SACB Inputs.IPS PartPresenceBottom LH"=w192:bool)
                  n69 = And(x=w191, y=w192) -> (x .and. y?=w190:bool)
                }
                frame "W 501 FRH Std.", "W 601 FR RH Std", "W 601 RR RH Std", "W 601 FR RH AP", "W 601 RR RH AP" {
                  n70 = Unbundle By Name(w197) -> ("SACB Inputs.IPS PartPresenceTop RH"=w195:bool, "SACB Inputs.IPS PartPresenceBottom RH"=w196:bool)
                  n71 = And(x=w195, y=w196) -> (x .and. y?=w194:bool)
                }
              }
              n72 = global read "Test auto state machine.vi" "Cluster"() -> (w180:T19)
              n73 = Unbundle By Name(w180) -> ("Part Presence"=w179:bool)
              n74 = Select(t=Auto_States_v0.2."Wait for Hands-Off", s=w179, f=Auto_States_v0.2."Wait for Part Presence") -> (s? t:f=w187:T7)
            }
            frame "Wait for Hands-Off" {
              n75 = Unbundle By Name(w202) -> ()  [unwired: 1 out]
              n76 = global read "Test auto state machine.vi" "Cluster"() -> (w199:T19)
              n77 = Unbundle By Name(w199) -> ("Hands Off"=w198:bool)
              n78 = Select(t=Auto_States_v0.2."Clamp", s=w198, f=Auto_States_v0.2."Wait for Hands-Off") -> (s? t:f=w203:T7)
            }
            frame "Clamp" {
              n79 = Unbundle By Name(w214) -> ("Model Name"=w213:T8)
              n80 = global read "Test auto state machine.vi" "Cluster"() -> (w208:T19)
              n81 = call "Clamp.vi"("Model Name"=w213, "Error In"=w216, "Intialize?"=w217, "Inputs"=w215) -> ("error out"=w211:errorcluster, "Completed"=w209:bool)  [unwired: 5 in, 1 out]
              n82 = Unbundle By Name(w208) -> ("Clamp"=w207:bool)
              n83 = case shown="No Error" w211 {
                tunnel: [w220 Auto_States_v0.2."Initialize"] -> w218
                tunnel: w209 -> [_ _]
                tunnel: w207 -> [w219 _]
                frame No Error {
                  n84 = Select(t=Auto_States_v0.2."Wait for Load Engage", s=w219, f=Auto_States_v0.2."Clamp") -> (s? t:f=w220:T7)
                }
                frame Error {
                }
              }
            }
            frame "Wait for Load Engage" {
              n85 = case shown="\"W 601 FR LH Std\", \"W 601 RR LH Std\", \"W 601 FR LH AP\", \"W 601 RR LH AP\"" w226 {
                tunnel: w229 -> [w237 w242 w244]
                tunnel: [w234 w240 w245] -> _
                frame "W 501 FLH Std.", "W 501 FRH Std." {
                  n86 = Unbundle By Name(w237) -> ("SACB Inputs.IPS LoadEngaged 1"=w236:bool, "SACB Inputs.IPS LoadEngaged 2"=w235:bool)
                  n87 = And(x=w236, y=w235) -> (x .and. y?=w234:bool)
                }
                frame "W 601 FR RH Std", "W 601 RR RH Std", "W 601 FR RH AP", "W 601 RR RH AP" {
                  n88 = Unbundle By Name(w242) -> ("SACB Inputs.IPS LoadEngaged 1"=w241:bool, "SACB Inputs.IPS LoadEngaged 2"=w239:bool, "SACB Inputs.IPS LoadEngaged 3"=w238:bool)
                  n89 = Compound Arithmetic op=AND(invert w241, w239, w238) -> (w240:bool)
                }
                frame "W 601 FR LH Std", "W 601 RR LH Std", "W 601 FR LH AP", "W 601 RR LH AP" {
                  n90 = Unbundle By Name(w244) -> ("SACB Inputs.IPS LoadEngaged 1"=w246:bool, "SACB Inputs.IPS LoadEngaged 2"=w247:bool, "SACB Inputs.IPS LoadEngaged 3"=w243:bool)
                  n91 = Compound Arithmetic op=AND(w246, invert w247, w243) -> (w245:bool)
                }
              }
              n92 = global read "Test auto state machine.vi" "Cluster"() -> (w225:T19)
              n93 = Unbundle By Name(w225) -> ("Load engage"=w224:bool)
              n94 = Select(t=Auto_States_v0.2."Wait for Start", s=w224, f=Auto_States_v0.2."Wait for Load Engage") -> (s? t:f=w232:T7)
            }
            frame "Wait for Start" {
              w248 = TRUE
              n95 = Unbundle By Name(w254) -> ("DI.E-Stop"=w261:bool, "DI.Safety Curtain"=w257:bool, "DI.Machine ON"=w260:bool, "DI.Door SW Reject"=w255:bool)
              n96 = Unbundle By Name(w259) -> ("Model Name"=w253:T8)
              n97 = global read "Test auto state machine.vi" "Cluster"() -> (w250:T19)
              n98 = Unbundle By Name(w254) -> ("DI.Start"=w251:bool)
              n99 = Unbundle By Name(w250) -> ("Wait Start"=w249:bool)
              n100 = case shown="\"W 501 FLH Std.\", \"W 601 FR LH Std\", \"W 601 RR LH Std\", \"W 601 FR LH AP\", \"W 601 RR LH AP\"" w253 {
                tunnel: w254 -> [w268 w272]
                tunnel: [w265 w269] -> w252
                frame "W 501 FLH Std.", "W 601 FR LH Std", "W 601 RR LH Std", "W 601 FR LH AP", "W 601 RR LH AP" {
                  n101 = Unbundle By Name(w268) -> ("SACB Inputs.IPS PartPresenceTop LH"=w266:bool, "SACB Inputs.IPS PartPresenceBottom LH"=w267:bool)
                  n102 = And(x=w266, y=w267) -> (x .and. y?=w265:bool)
                }
                frame "W 501 FRH Std.", "W 601 FR RH Std", "W 601 RR RH Std", "W 601 FR RH AP", "W 601 RR RH AP" {
                  n103 = Unbundle By Name(w272) -> ("SACB Inputs.IPS PartPresenceTop RH"=w270:bool, "SACB Inputs.IPS PartPresenceBottom RH"=w271:bool)
                  n104 = And(x=w270, y=w271) -> (x .and. y?=w269:bool)
                }
              }
              n105 = Compound Arithmetic op=AND(w251, w257) -> (w258:bool)
              n106 = Compound Arithmetic op=AND(w261, w260, w252, w255) -> ()  [unwired: 1 out]
              n107 = case shown="True" w248 {
                tunnel: w258 -> [_ _]
                tunnel: [Auto_States_v0.2."Initialize" w277] -> w264
                tunnel: w249 -> [_ w276]
                frame False {
                  n108 = call "FGV - DO.vi"("Digital Outs"=bool[] [FALSE, FALSE, FALSE, FALSE], "State"=FGV_DO."Clamping") -> ()  [unwired: 8 in, 2 out]
                }
                frame True {
                  n109 = Select(t=Auto_States_v0.2."Test Sequencer", s=w276, f=Auto_States_v0.2."Wait for Start") -> (s? t:f=w277:T7)
                }
              }
              n110 = Tick Count (ms)() -> (millisecond timer value=w256:u32)
            }
            frame "Test Sequencer" {
              n111 = call "Test Sequencer.vi"("Initial Data"=w281, "Error In"=w301, "Initialize"=w300, "Inputs"=w289) -> ("Error Out"=w294:errorcluster, "Completed?"=w290:bool, "Results"=w288:T1, "Results Cluster out"=w287:T2, "Graph"=→"Graph 2":dbl[][], "TS Status"=→"TS Status 2":cluster{"Status":string, "Elapsed Time":dbl})  [unwired: 2 in]
              "Results Cluster out 2" <- w287
              n112 = call "Pass-Fail.vi"("Counts in"=w292, "error in"=w294, "Completed? in"=w290, "Results in"=w288, "Results Cluster in"=w287) -> ("error out"=w293:errorcluster, "Completed? out"=w280:bool, "Results out"=→"Results 2":T1, "Counts out"=w291:T6)  [unwired: 3 in]
              n113 = Tick Count (ms)() -> (millisecond timer value=w284:u32)
              n114 = global write "Towerlight GV.vi" "Status"(Towerlight."Running" ("Status")) -> ()
              n115 = Subtract(x=w284, y=w282) -> (x-y=→"cycle time 2":u32)
              n116 = Select(t=Auto_States_v0.2."Log & Print", s=w280, f=Auto_States_v0.2."Test Sequencer") -> (s? t:f=w297:T7)
            }
            frame "Log & Print" {
              # "Change needed here"
              # "0- <Name in>\n1- <Common Name>\n \n2- Part No\n3- Name\n4- ID\n5- DATE-Time"
              n117 = local read "Results 2"() -> (w320:T1)
              n118 = Unbundle By Name(w328) -> ("Model Name"=w319:T8, "ID"=w324:string, "Shift"=w302:string)
              n119 = Unbundle By Name(w313) -> ("TotalCount"=w312:u16)
              n120 = case shown="\"W 501 FRH Std.\"" w319 {
                tunnel: [string[] ["", "", "0111HW500041N", "WR ASSY FRH W501"] ("PrintPara") string[] ["", "", "0111HW500051N", "WR ASSY FLH W501"] ("PrintPara") string[] ["", "", "0111HW500041N", "WR ASSY FR RH W601"] ("PrintPara") string[] ["", "", "0111HW500041N", "WR ASSY FR LH W601"] ("PrintPara") string[] ["", "", "0111HW500041N", "WR ASSY RR RH W601"] ("PrintPara") string[] ["", "", "0111HW500041N", "WR ASSY RR LH W601"] ("PrintPara") string[] ["", "", "0111HW500041N", "WR ASSY FR RH AP W601"] ("PrintPara") string[] ["", "", "0111HW500041N", "WR ASSY FR LH AP W601"] ("PrintPara") string[] ["", "", "0111HW500041N", "WR ASSY RR RH AP W601"] ("PrintPara") string[] ["", "", "0111HW500041N", "WR ASSY RR LH AP W601"] ("PrintPara")] -> w323
                frame "W 501 FRH Std." {
                }
                frame "W 501 FLH Std." {
                }
                frame "W 601 FR RH Std" {
                }
                frame "W 601 FR LH Std" {
                }
                frame "W 601 RR RH Std" {
                }
                frame "W 601 RR LH Std" {
                }
                frame "W 601 FR RH AP" {
                }
                frame "W 601 FR LH AP" {
                }
                frame "W 601 RR RH AP" {
                }
                frame "W 601 RR LH AP" {
                }
              }
              n121 = Unbundle By Name(w320) -> ("Initial.Date"=w304:string, "Initial.Time"=w303:string, "Results.PASS?"=w315:bool)
              n122 = call "Write Datalog.vi"("error in"=w318, "Model Name"=w319, "Results"=w320, "file path (dialog if empty)"=w321) -> ("error in"=w317:errorcluster)  [unwired: 7 in]
              n123 = Insert Into Array(array=w323, index=4, new element #1=w324, new element #2=w302) -> (w326:string[])
              n124 = Format Into String(w312) -> (resulting string=w310:string)  [unwired: 3 in, 1 out]
              n125 = Insert Into Array(array=w326, index=6, new element #1=w304, new element #2=w303) -> (w308:string[])
              n126 = Concatenate Strings(w304, "" ("string"), w303) -> ()  [unwired: 1 out]
              n127 = Concatenate Strings(w310, "     " ("string"), "OK" ("string")) -> (w305:string)
              n128 = Insert Into Array(array=w308, index=8, new element=w305) -> (w307:string[])
              n129 = case shown="True" w315 {
                tunnel: w307 -> [_ w329]
                frame False {
                }
                frame True {
                  n130 = call "PrintLabel v0.4.vi"("PrintPara"=w329) -> ()  [unwired: 10 in, 1 out]
                }
              }
            }
            frame "Result" {
              # "Part Removed?"
              n131 = local read "Results 2"() -> (w342:T1)
              n132 = Unbundle By Name(w349) -> ("Model Name"=w346:T8)
              n133 = Unbundle By Name(w345) -> ("DI.Safety Curtain"=w344:bool)
              n134 = case shown="\"W 501 FLH Std.\"" w346 {
                tunnel: w345 -> [w360 w361 w368 w372 w376 w380 w384 w388 w392 w396]
                tunnel: [w357 w363 w365 w369 w373 w377 w381 w385 w389 w393] -> w343
                frame "W 501 FLH Std." {
                  n135 = Unbundle By Name(w360) -> ("SACB Inputs.IPS PartPresenceTop LH"=w359:bool, "SACB Inputs.IPS PartPresenceBottom LH"=w358:bool)
                  n136 = Compound Arithmetic op=AND(invert w359, invert w358) -> (w357:bool)
                }
                frame "W 501 FRH Std." {
                  n137 = Unbundle By Name(w361) -> ("SACB Inputs.IPS PartPresenceTop RH"=w364:bool, "SACB Inputs.IPS PartPresenceBottom RH"=w362:bool)
                  n138 = Compound Arithmetic op=AND(invert w364, invert w362) -> (w363:bool)
                }
                frame "W 601 FR RH Std" {
                  n139 = Unbundle By Name(w368) -> ("SACB Inputs.IPS PartPresenceTop RH"=w367:bool, "SACB Inputs.IPS PartPresenceBottom RH"=w366:bool)
                  n140 = Compound Arithmetic op=AND(invert w367, invert w366) -> (w365:bool)
                }
                frame "W 601 FR LH Std" {
                  n141 = Unbundle By Name(w372) -> ("SACB Inputs.IPS PartPresenceTop LH"=w371:bool, "SACB Inputs.IPS PartPresenceBottom LH"=w370:bool)
                  n142 = Compound Arithmetic op=AND(invert w371, invert w370) -> (w369:bool)
                }
                frame "W 601 RR RH Std" {
                  n143 = Unbundle By Name(w376) -> ("SACB Inputs.IPS PartPresenceTop RH"=w375:bool, "SACB Inputs.IPS PartPresenceBottom RH"=w374:bool)
                  n144 = Compound Arithmetic op=AND(invert w375, invert w374) -> (w373:bool)
                }
                frame "W 601 RR LH Std" {
                  n145 = Unbundle By Name(w380) -> ("SACB Inputs.IPS PartPresenceTop LH"=w379:bool, "SACB Inputs.IPS PartPresenceBottom LH"=w378:bool)
                  n146 = Compound Arithmetic op=AND(invert w379, invert w378) -> (w377:bool)
                }
                frame "W 601 FR RH AP" {
                  n147 = Unbundle By Name(w384) -> ("SACB Inputs.IPS PartPresenceTop RH"=w383:bool, "SACB Inputs.IPS PartPresenceBottom RH"=w382:bool)
                  n148 = Compound Arithmetic op=AND(invert w383, invert w382) -> (w381:bool)
                }
                frame "W 601 FR LH AP" {
                  n149 = Unbundle By Name(w388) -> ("SACB Inputs.IPS PartPresenceTop LH"=w387:bool, "SACB Inputs.IPS PartPresenceBottom LH"=w386:bool)
                  n150 = Compound Arithmetic op=AND(invert w387, invert w386) -> (w385:bool)
                }
                frame "W 601 RR RH AP" {
                  n151 = Unbundle By Name(w392) -> ("SACB Inputs.IPS PartPresenceTop RH"=w391:bool, "SACB Inputs.IPS PartPresenceBottom RH"=w390:bool)
                  n152 = Compound Arithmetic op=AND(invert w391, invert w390) -> (w389:bool)
                }
                frame "W 601 RR LH AP" {
                  n153 = Unbundle By Name(w396) -> ("SACB Inputs.IPS PartPresenceTop LH"=w395:bool, "SACB Inputs.IPS PartPresenceBottom LH"=w394:bool)
                  n154 = Compound Arithmetic op=AND(invert w395, invert w394) -> (w393:bool)
                }
              }
              n155 = Unbundle By Name(w342) -> ("Results.PASS?"=w340:bool)
              n156 = Compound Arithmetic op=AND(w344, w343) -> (w341:bool)
              n157 = case shown="True" w341 {
                tunnel: [Auto_States_v0.2."Result" w354] -> w351
                tunnel: w340 -> [_ w353]
                frame False {
                }
                frame True {
                  n158 = Select(t=Auto_States_v0.2."Initialize", s=w353, f=Auto_States_v0.2."Wait for Reject Door Open") -> (s? t:f=w354:T7)
                }
              }
            }
            frame "Wait for Reject Door Open" {
              n159 = Unbundle By Name(w398) -> ("DI.Door SW Reject"=w397:bool)
              n160 = disable-structure shown="Disabled" {
                frame Disabled {
                  n161 = global write "Towerlight GV.vi" "Status"(Towerlight."Fail" ("Status")) -> ()
                }
                frame Enabled {
                }
              }
              n162 = Select(t=Auto_States_v0.2."Wait for Reject Door Open", s=w397, f=Auto_States_v0.2."Wait for Reject 2 OFF") -> (s? t:f=w403:T7)
            }
            frame "Wait for Reject 2 OFF" {
              n163 = Unbundle By Name(w407) -> ("DI.Reject Sensor 2"=w406:bool)
              n164 = Select(t=Auto_States_v0.2."Wait for Reject 2 OFF", s=w406, f=Auto_States_v0.2."Wait for Reject 2 ON") -> (s? t:f=w412:T7)
            }
            frame "Wait for Reject 2 ON" {
              n165 = Unbundle By Name(w415) -> ("DI.Reject Sensor 2"=w414:bool)
              n166 = Select(t=Auto_States_v0.2."Wait for Reject 1 OFF", s=w414, f=Auto_States_v0.2."Wait for Reject 2 ON") -> (s? t:f=w420:T7)
            }
            frame "Wait for Reject 1 OFF" {
              n167 = Unbundle By Name(w423) -> ("DI.Reject Sensor 1"=w422:bool)
              n168 = Select(t=Auto_States_v0.2."Wait for Reject 1 OFF", s=w422, f=Auto_States_v0.2."Wait for Reject 1 ON") -> (s? t:f=w428:T7)
            }
            frame "Wait for Reject 1 ON" {
              n169 = Unbundle By Name(w431) -> ("DI.Reject Sensor 1"=w430:bool)
              n170 = Select(t=Auto_States_v0.2."Wait for Reject Door Close", s=w430, f=Auto_States_v0.2."Wait for Reject 1 ON") -> (s? t:f=w436:T7)
            }
            frame "Wait for Reject Door Close" {
              n171 = Unbundle By Name(w447) -> ("DI.Reject Sensor 1"=w446:bool, "DI.Reject Sensor 2"=w445:bool, "DI.Door SW Reject"=w442:bool)
              n172 = Not(x=w446) -> (.not. x?=w441:bool)
              n173 = Not(x=w445) -> (.not. x?=w440:bool)
              n174 = Build Array(w441, w440, w442) -> (w444:bool[])
              n175 = Search 1D Array(1D array=w444, element=TRUE) -> ()  [unwired: 1 in, 1 out]
              n176 = case shown="2" 2 {
                tunnel: [Auto_States_v0.2."Wait for Reject 1 ON" Auto_States_v0.2."Wait for Reject Door Close" Auto_States_v0.2."Wait for Reject 2 ON" Auto_States_v0.2."Initialize"] -> w439
                frame 0, Default {
                  # "reject 1 has been cut"
                }
                frame -1 {
                  # "None of the booleans have become TRUE"
                }
                frame 1 {
                  # "reject 2 has been cut"
                }
                frame 2 {
                  # "Correct procedure, door is closed"
                }
              }
            }
          }
          "AC State" <- w76
          "Counts" <- w70
          n177 = Unbundle By Name(w61) -> ("status"=w60:bool)
          n178 = Compound Arithmetic op=OR("Run Auto?") -> (w80:bool)
          n179 = Select(t=Towerlight."Error" ("Status"), s=w60, f=Towerlight."Idle" ("Status")) -> (s? t:f=w58:T12)
          n180 = node-c288() -> ()  [unwired: 1 in, 1 out]
          n181 = global write "Towerlight GV.vi" "Status"(w58) -> ()
        }
        n182 = node-c288(w51) -> ()  [unwired: 1 out]
      }
    }
  }
  n183 = while {
    tunnel: w12 -> [w465]
    tunnel: "error in" -> [w470]
    tunnel: [w464] -> w11
    tunnel: w9 -> [w463]
    stop <- w468 stop-if-true
    n184 = call "Dequeue Message.vi"("timeout"=100, "error in (no error)"=w470, "Message Queue"=w465) -> ("error out"=w471:errorcluster, "Message Data"=w472:variant, "Message"=w474:string, "dup Message Queue"=w473:refnum<queue>)  [unwired: 5 in]
    n185 = case shown="\"Timeout\"" w474 {
      selector: w474 -> [_ _ _ _ _ w523 _]
      tunnel: w473 -> [_ _ _ _ _ _ w532]
      tunnel: w472 -> [w480 w488 _ _ w519 _ _]
      tunnel: w471 -> [w482 w489 w494 w512 w518 w529 w531]
      tunnel: [w481 w487 w493 w512 w516 w528 w530] -> w464
      tunnel: [_ _ _ _ _ _ w533] -> w468
      tunnel: w463 -> [_ _ w492 _ w514 w527 _]
      frame "Start Auto Mode" {
        n186 = Variant To Data(error in=w482, type=T9 {"Model Name"=enum."W 501 FLH Std.", "ID"="ID", "Shift"=""} ("Initial Data 2"), Variant=w480) -> (data=w478:T9, error out=w481:errorcluster)
        n187 = local write "Initial Data"(w478) -> ()
        n188 = flat-sequence {
          tunnel: w478 -> [_]
          frame #0 {
            n189 = Wait (ms)(milliseconds to wait=u32 100) -> ()  [unwired: 1 out]
          }
          frame #1 {
            n190 = local write "Run Auto?"(TRUE ("Stop Test")) -> ()
          }
        }
      }
      frame "Update Specs" {
        n191 = Variant To Data(error in=w489, type=T4 {"LH"={"Go Up"={"Min Speed"=120.0, "Max Speed"=10.0, "Min Time"=1.82, "Max Time"=3.7, "Min Run Current"=0.0, "Max Run Current"=10.0, "Min Stall Current"=0.0, "Max Stall Current"=25.0, "Min Stall Force"=170.0, "Max Stall Force"=320.0, "Min Stroke"=170.0, "Max Stroke"=320.0}, "Go Down"={"Min Speed"=10.0, "Max Speed"=250.0, "Min Travel Time"=1.82, "Max Travel Time"=3.7, "Min Run Current"=0.0, "Max Run Current"=10.0}, "Shipping"={"Min Distance"=150.0, "Max Distance"=300.0, "Setpoint"=5.0}, "Anti-Pinch"={"Min Force"=5.0, "Max Force"=15.0}}, "RH"={"Go Up"={"Min Speed"=120.0, "Max Speed"=10.0, "Min Time"=1.82, "Max Time"=3.7, "Min Run Current"=0.0, "Max Run Current"=10.0, "Min Stall Current"=0.0, "Max Stall Current"=25.0, "Min Stall Force"=170.0, "Max Stall Force"=320.0, "Min Stroke"=170.0, "Max Stroke"=320.0}, "Go Down"={"Min Speed"=10.0, "Max Speed"=250.0, "Min Travel Time"=1.82, "Max Travel Time"=3.7, "Min Run Current"=0.0, "Max Run Current"=10.0}, "Shipping"={"Min Distance"=150.0, "Max Distance"=300.0, "Setpoint"=5.0}, "Anti-Pinch"={"Min Force"=5.0, "Max Force"=15.0}}, "W 601 FR RH Std"={"Go Up"={"Min Speed"=10.0, "Max Speed"=250.0, "Min Time"=0.5, "Max Time"=4.3, "Min Run Current"=0.0, "Max Run Current"=10.0, "Min Stall Current"=0.0, "Max Stall Current"=25.0, "Min Stall Force"=170.0, "Max Stall Force"=320.0, "Min Stroke"=254.4, "Max Stroke"=270.4}, "Go Down"={"Min Speed"=10.0, "Max Speed"=250.0, "Min Travel Time"=0.5, "Max Travel Time"=4.3, "Min Run Current"=0.0, "Max Run Current"=10.0}, "Shipping"={"Min Distance"=5.0, "Max Distance"=15.0, "Setpoint"=5.0}, "Anti-Pinch"={"Min Force"=5.0, "Max Force"=15.0}}, "W 601 FR LH Std"={"Go Up"={"Min Speed"=10.0, "Max Speed"=250.0, "Min Time"=0.5, "Max Time"=4.3, "Min Run Current"=0.0, "Max Run Current"=10.0, "Min Stall Current"=0.0, "Max Stall Current"=25.0, "Min Stall Force"=170.0, "Max Stall Force"=320.0, "Min Stroke"=254.4, "Max Stroke"=270.4}, "Go Down"={"Min Speed"=10.0, "Max Speed"=250.0, "Min Travel Time"=0.5, "Max Travel Time"=4.3, "Min Run Current"=0.0, "Max Run Current"=10.0}, "Shipping"={"Min Distance"=5.0, "Max Distance"=15.0, "Setpoint"=5.0}, "Anti-Pinch"={"Min Force"=5.0, "Max Force"=15.0}}, "W 601 RR RH Std"={"Go Up"={"Min Speed"=10.0, "Max Speed"=250.0, "Min Time"=0.5, "Max Time"=4.3, "Min Run Current"=0.0, "Max Run Current"=10.0, "Min Stall Current"=0.0, "Max Stall Current"=25.0, "Min Stall Force"=170.0, "Max Stall Force"=320.0, "Min Stroke"=254.4, "Max Stroke"=270.4}, "Go Down"={"Min Speed"=10.0, "Max Speed"=250.0, "Min Travel Time"=0.5, "Max Travel Time"=4.3, "Min Run Current"=0.0, "Max Run Current"=10.0}, "Shipping"={"Min Distance"=5.0, "Max Distance"=15.0, "Setpoint"=5.0}, "Anti-Pinch"={"Min Force"=5.0, "Max Force"=15.0}}, "W 601 RR LH Std"={"Go Up"={"Min Speed"=10.0, "Max Speed"=250.0, "Min Time"=0.5, "Max Time"=4.3, "Min Run Current"=0.0, "Max Run Current"=10.0, "Min Stall Current"=0.0, "Max Stall Current"=25.0, "Min Stall Force"=170.0, "Max Stall Force"=320.0, "Min Stroke"=254.4, "Max Stroke"=270.4}, "Go Down"={"Min Speed"=10.0, "Max Speed"=250.0, "Min Travel Time"=0.5, "Max Travel Time"=4.3, "Min Run Current"=0.0, "Max Run Current"=10.0}, "Shipping"={"Min Distance"=5.0, "Max Distance"=15.0, "Setpoint"=5.0}, "Anti-Pinch"={"Min Force"=5.0, "Max Force"=15.0}}, "W 601 FR RH AP"={"Go Up"={"Min Speed"=10.0, "Max Speed"=250.0, "Min Time"=0.5, "Max Time"=4.3, "Min Run Current"=0.0, "Max Run Current"=10.0, "Min Stall Current"=0.0, "Max Stall Current"=25.0, "Min Stall Force"=170.0, "Max Stall Force"=320.0, "Min Stroke"=254.4, "Max Stroke"=270.4}, "Go Down"={"Min Speed"=10.0, "Max Speed"=250.0, "Min Travel Time"=0.5, "Max Travel Time"=4.3, "Min Run Current"=0.0, "Max Run Current"=10.0}, "Shipping"={"Min Distance"=5.0, "Max Distance"=15.0, "Setpoint"=5.0}, "Anti-Pinch"={"Min Force"=5.0, "Max Force"=15.0}}, "W 601 FR LH AP"={"Go Up"={"Min Speed"=10.0, "Max Speed"=250.0, "Min Time"=0.5, "Max Time"=4.3, "Min Run Current"=0.0, "Max Run Current"=10.0, "Min Stall Current"=0.0, "Max Stall Current"=25.0, "Min Stall Force"=170.0, "Max Stall Force"=320.0, "Min Stroke"=254.4, "Max Stroke"=270.4}, "Go Down"={"Min Speed"=10.0, "Max Speed"=250.0, "Min Travel Time"=0.5, "Max Travel Time"=4.3, "Min Run Current"=0.0, "Max Run Current"=10.0}, "Shipping"={"Min Distance"=5.0, "Max Distance"=15.0, "Setpoint"=5.0}, "Anti-Pinch"={"Min Force"=5.0, "Max Force"=15.0}}, "W 601 RR RH AP"={"Go Up"={"Min Speed"=10.0, "Max Speed"=250.0, "Min Time"=0.5, "Max Time"=4.3, "Min Run Current"=0.0, "Max Run Current"=10.0, "Min Stall Current"=0.0, "Max Stall Current"=25.0, "Min Stall Force"=170.0, "Max Stall Force"=320.0, "Min Stroke"=254.4, "Max Stroke"=270.4}, "Go Down"={"Min Speed"=10.0, "Max Speed"=250.0, "Min Travel Time"=0.5, "Max Travel Time"=4.3, "Min Run Current"=0.0, "Max Run Current"=10.0}, "Shipping"={"Min Distance"=5.0, "Max Distance"=15.0, "Setpoint"=5.0}, "Anti-Pinch"={"Min Force"=5.0, "Max Force"=15.0}}, "W 601 RR LH AP"={"Go Up"={"Min Speed"=10.0, "Max Speed"=250.0, "Min Time"=0.5, "Max Time"=4.3, "Min Run Current"=0.0, "Max Run Current"=10.0, "Min Stall Current"=0.0, "Max Stall Current"=25.0, "Min Stall Force"=170.0, "Max Stall Force"=320.0, "Min Stroke"=254.4, "Max Stroke"=270.4}, "Go Down"={"Min Speed"=10.0, "Max Speed"=250.0, "Min Travel Time"=0.5, "Max Travel Time"=4.3, "Min Run Current"=0.0, "Max Run Current"=10.0}, "Shipping"={"Min Distance"=5.0, "Max Distance"=15.0, "Setpoint"=5.0}, "Anti-Pinch"={"Min Force"=5.0, "Max Force"=15.0}}} ("All Specs"), Variant=w488) -> (data=→"Specs":T4, error out=w487:errorcluster)
      }
      frame "Timeout" {
        # "Update all Indicators"
        n192 = local read "AC State"() -> (w490:T7)
        n193 = local read "Run Auto?"() -> (w491:bool)
        n194 = case shown="True" w491 {
          tunnel: w492 -> [w509 _]
          tunnel: w494 -> [w508 w510]
          tunnel: [w503 w510] -> w493
          tunnel: w490 -> [w502 _]
          frame True {
            n195 = local read "cycle time 2"() -> (w495:u32)
            n196 = call-poly "Enqueue Message.vi"("error in (no error)"=w508, "Message Data"=w502, "Message"="Update Status", "Message Queue"=w509) -> ("error out"=w504:errorcluster, "dup Message Queue"=w505:refnum<queue>)  [unwired: 6 in]
            n197 = local read "Counts"() -> (w498:T6)
            n198 = local read "Graph 2"() -> (w496:dbl[][])
            n199 = local read "TS Status 2"() -> (w501:cluster{"Status":string, "Elapsed Time":dbl})
            n200 = local read "Results 2"() -> (w497:T1)
            n201 = Bundle(cluster=T20 {"Results"={"Initial"={"Date"="", "Time"="", "ID"=""}, "Go Up"={"Speed"=0.0, "Travel Time"=0.0, "Running Current"=0.0, "Up Stroke"=0.0, "Stall Current"=0.0, "Stall Force"=0.0}, "Go Down"={"Speed"=0.0, "Travel Time"=0.0, "Running Current"=0.0, "Down Stroke"=0.0}, "Shipping Position"={"Shipping Position"=0.0}, "Results"={"PASS?"=FALSE, "Details"=""}, "Antipinch"={"Pinch Force"=0.0}}, "TS Status"={"Status"="", "Elapsed Time"=0.0}, "Counts"={"TotalCount"=0, "PassCount"=0, "FailCount"=0}, "AC Graph"=[], "Total Time"=0.0, "Testing Time (s)"=0.0, "Graph"=[], "signal out"={"t0"=timestamp(0 s since 1904-01-01), "dt"=1.0, "Y"=[]}}, "Results"=w497, "TS Status"=w501, "Counts"=w498, "Testing Time (s)"=w495, "Graph"=w496) -> (w500:T20)  [unwired: 3 in]
            n202 = call-poly "Enqueue Message.vi"("error in (no error)"=w504, "Message Data"=w500, "Message"="Update Measurements", "Message Queue"=w505) -> ("error out"=w503:errorcluster)  [unwired: 6 in, 1 out]
          }
          frame False {
          }
        }
      }
      frame "End Auto Mode" {
        n203 = local write "Run Auto?"(FALSE ("Stop Test")) -> ()
      }
      frame "Error" {
        n204 = Variant To Data(error in=w518, type=w518, Variant=w519) -> (data=w515:errorcluster, error out=w517:errorcluster)
        n205 = call-poly "Enqueue Message.vi"("error in (no error)"=w517, "Message Data"=w515, "Message"="Error", "Message Queue"=w514) -> ("error out"=w516:errorcluster)  [unwired: 6 in, 1 out]
      }
      frame Default {
        n206 = Concatenate Strings("Unknown or prohibited command received: " ("source"), w523) -> (w522:string)
        n207 = Bundle(cluster=errorcluster {"status"=FALSE, "code"=0, "source"=""} ("error constant"), "code"=5010, "source"=w522) -> (w520:errorcluster)  [unwired: 1 in]
        n208 = call-poly "Enqueue Message.vi"("error in (no error)"=w529, "Message Data"=w520, "Message"="Error", "Message Queue"=w527) -> ("error out"=w528:errorcluster)  [unwired: 6 in, 1 out]
      }
      frame "Exit" {
        w533 = TRUE ("Stop Test")
        n209 = Release Queue(queue=w532, error in (no error)=w531) -> (error out=w530:errorcluster)  [unwired: 1 in, 2 out]
        n210 = local write "Run Auto?"(FALSE ("Stop Test")) -> ()
        n211 = local write "Exit"(w533) -> ()
      }
    }
    n212 = Merge Errors(w464) -> (w467:errorcluster)
    n213 = Unbundle By Name(w467) -> ("code"=w466:i32)
    n214 = case shown="Default" w466 {
      tunnel: w465 -> [_ w477]
      tunnel: w464 -> [_ w475]
      frame 0 {
        # "All OK"
      }
      frame Default {
        n215 = call-poly "Enqueue Message.vi"("Message Data"=w475, "Message"="Error", "Message Queue"=w477) -> ()  [unwired: 7 in, 2 out]
      }
    }
  }
  n216 = call "Auto Stop Tasks.vi"("error in"=w3, "All Input Tasks in"=w5) -> ("error out"=w4:errorcluster)  [unwired: 9 in]
  n217 = Merge Errors(w4, w11) -> (→"error out":errorcluster)
  "semaphore out" <- "semaphore"
